vi "Phasor Explorer SEPL Plot Name.vi"(8 "Error In":errorcluster, 11 "Phasor Parameters":T1 {"Detector Parameters"."Frames/Image" min=1; "Detector Parameters"."Multiplicity" min=0; "Detector Parameters"."Bits/Frame" min=1; "Detector Parameters"."Gates/Frame" min=1; "Gate Parameters"."# Steps" min=0.0; "Gate Parameters"."Tolerance" min=0.0; "Gate Parameters"."Top Slope" min=0.0; "Gate Parameters"."Edge Width" min=0.0; "Gate Parameters"."Gate Step" min=0.0; "Gate Parameters"."# Gates" min=0.0 step=1.0; "Gate Parameters"."Gate Width" min=0.0; "Decay & IRF Parameters"."Lifetime" min=0.0; "Decay & IRF Parameters"."IRF Period" min=0.0; "Phasor Parameters"."Square Gate Width" min=0.0; "Phasor Parameters"."# Gates" min=0.0; "Phasor Parameters"."Calibration Lifetime" min=0.0; "Phasor Parameters"."Harmonic Frequency" min=0.0; "Display Parameters"."Min tau" min=0.0; "Display Parameters"."Max tau" min=0.0; "Display Parameters"."# Points" min=1 step=1}) -> (0 "Error Out":errorcluster, 3 "SEPL Plot Name":string)   [LabVIEW 2021, in "Phasor Explorer.lvlib"]
uses:
  Phasor Explorer.lvlib
  Phasor SEPL Parameters.ctl
  Phasor Explorer Display Parameters.ctl
  Phasor Type of Series.ctl
  Phasor Explorer Phasor Parameters.ctl
  Phasor Calculation Type.ctl
  Phasor SEPL Type.ctl
  Phasor Explorer Decay Parameters.ctl
  Phasor IRF Model.ctl
  Phasor Explorer Gate Parameters.ctl
  Phasor Gate Type.ctl
  Phasor Type of User-defined Function.ctl
  Phasor Explorer Detector Parameters.ctl
  Phasor.lvlib
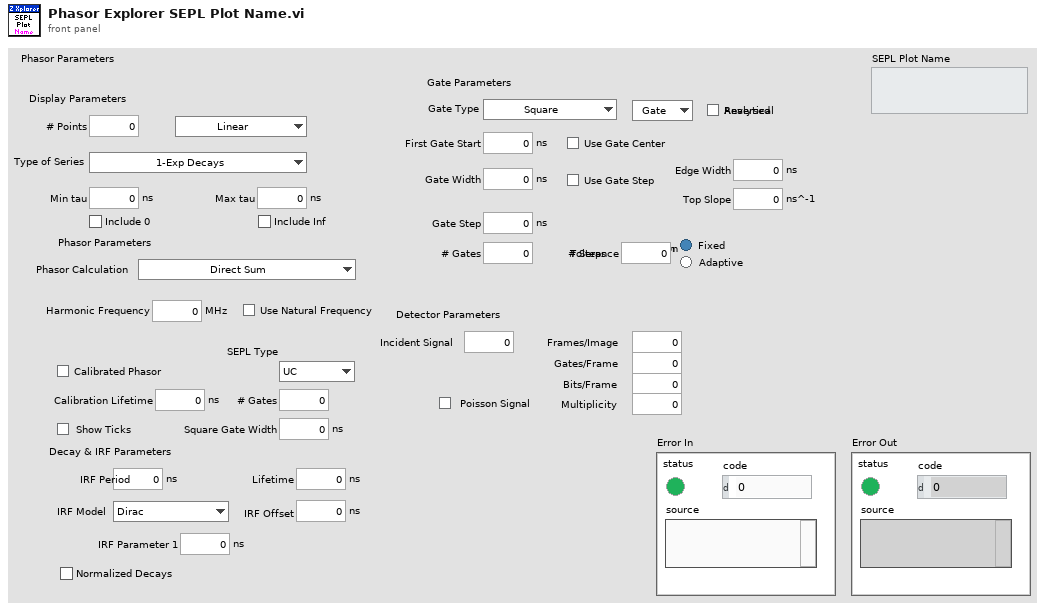
[diagram p1: front panel]
types:
  T1 = typedef "Phasor.lvlib/Phasor SEPL Parameters.ctl" = cluster{"Display Parameters":T2, "Phasor Parameters":T4, "Decay & IRF Parameters":T7, "Gate Parameters":T9, "Detector Parameters":T12}
  T2 = typedef "Phasor Explorer.lvlib/Phasor Explorer Display Parameters.ctl" = cluster{"# Points":i32, "Ramp Type":enum16{"Linear", "Logarithmic"}, "Type of Series":T3, "Min tau":dbl[unit], "Max tau":dbl[unit], "Include 0":bool, "Include Infinity":bool}
  T3 = typedef "Phasor.lvlib/Phasor Type of Series.ctl" = enum16{"1-Exp Decays", "Linear Combination of 1-Exp"}
  T4 = typedef "Phasor Explorer.lvlib/Phasor Explorer Phasor Parameters.ctl" = cluster{"Harmonic Frequency":dbl[unit], "Use f* = 1/D Frequency":bool, "Calibrated Phasor":bool, "Calibration Lifetime":dbl[unit], "Phasor Calculation":T5, "SEPL Type":T6, "# Gates":dbl, "Square Gate Width":dbl[unit], "Show Ticks":bool}
  T5 = typedef "Phasor.lvlib/Phasor Calculation Type.ctl" = enum16{"Direct Sum", "Analytical Formula"}
  T6 = typedef "Phasor.lvlib/Phasor SEPL Type.ctl" = enum16{"UC", "L_N", "L_N[W]", "L_X"}
  T7 = typedef "Phasor Explorer.lvlib/Phasor Explorer Decay Parameters.ctl" = cluster{"Lifetime":dbl[unit], "IRF Offset":dbl[unit], "IRF Period":dbl[unit], "Normalized Decays":bool, "IRF Model":T8, "IRF Parameter 1":dbl[unit]}
  T8 = typedef "Phasor.lvlib/Phasor IRF Model.ctl" = enum16{"Dirac", "Exponential"}
  T9 = typedef "Phasor Explorer.lvlib/Phasor Explorer Gate Parameters.ctl" = cluster{"First Gate Start":dbl[unit], "Use Gate Center":bool, "Gate Width":dbl[unit], "Gate Step":dbl[unit], "# Gates":dbl, "Gate Type":T10, "Edge Width":dbl[unit], "Top Slope":dbl[unit], "Reversed Sawtooth?":bool, "Analytical Computation":bool, "Integration":enum32{"Item 0", "Item 1"}, "Tolerance":dbl, "# Steps":dbl, "Type of User-defined Function":T11, "Use Gate Step":bool}
  T10 = typedef "Phasor.lvlib/Phasor Gate Type.ctl" = enum16{"Square", "Finite Edge Square", "Finite Edge, Tilted Top Square", "Triangle", "Sawtooth", "User-defined"}
  T11 = typedef "Phasor.lvlib/Phasor Type of User-defined Function.ctl" = enum16{"Gate", "IRF"}
  T12 = typedef "Phasor Explorer.lvlib/Phasor Explorer Detector Parameters.ctl" = cluster{"Frames/Image":i32, "Gates/Frame":i32, "Bits/Frame":i32, "Multiplicity":i32, "Incident Signal":dbl, "Poisson Signal":bool}
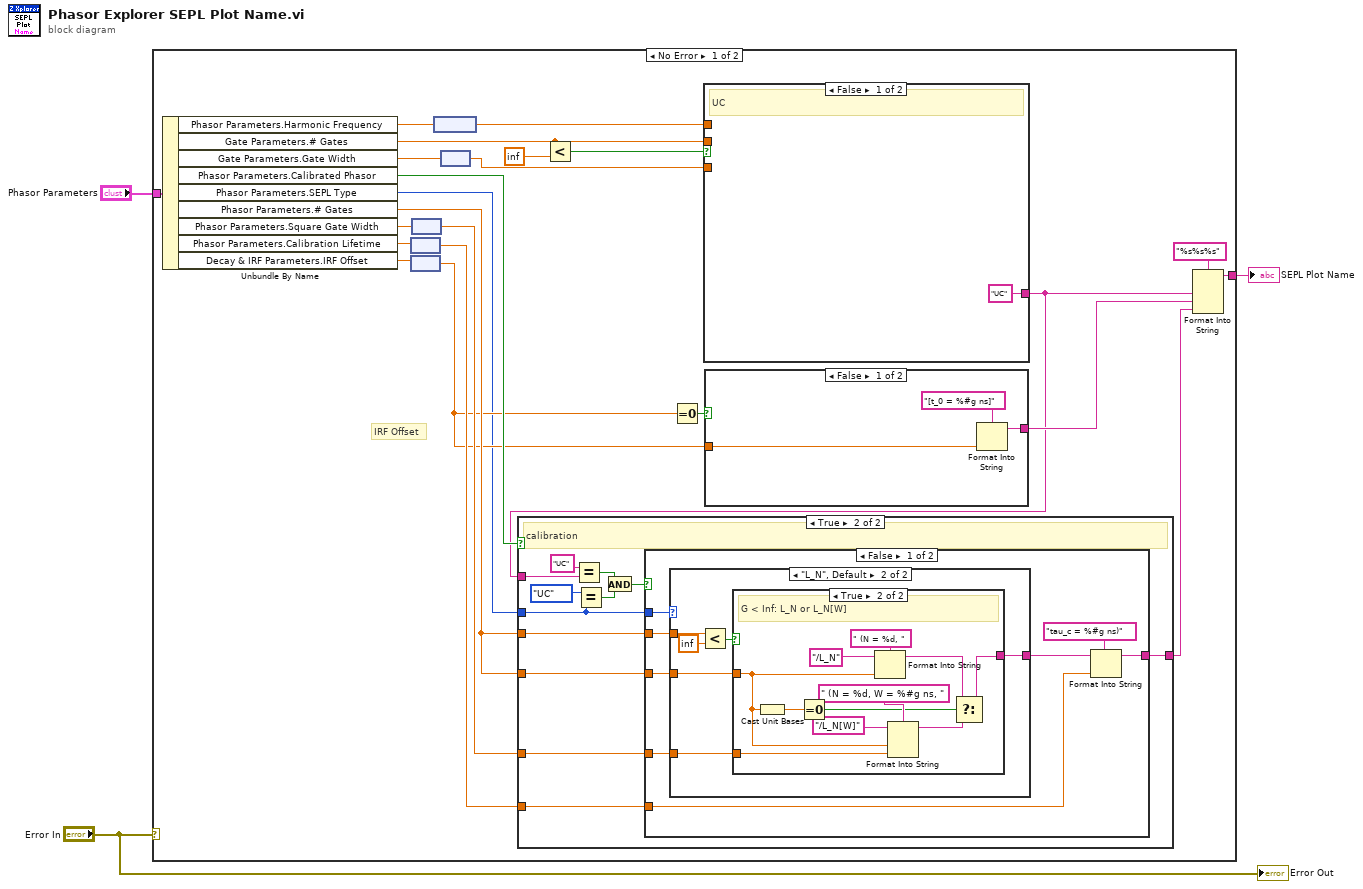
[diagram p0: block diagram]
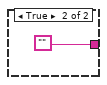
[diagram p2: hidden frame]
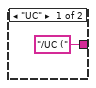
[diagram p4: hidden frame]
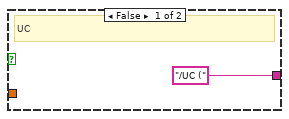
[diagram p5: hidden frame]
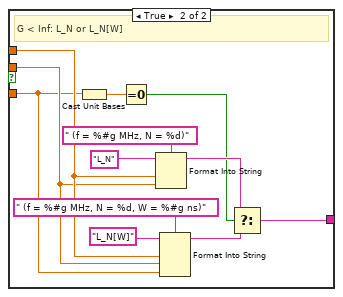
[diagram p7: hidden frame]
diagram:
  n1 = case shown="No Error" "Error In" {
    tunnel: "Phasor Parameters" -> [w25 _]
    tunnel: [w21 _] -> w2
    frame No Error {
      # "IRF Offset"
      n2 = Unbundle By Name(w25) -> ("Phasor Parameters.Harmonic Frequency"=w20:dbl[unit], "Gate Parameters.# Gates"=w19:dbl, "Gate Parameters.Gate Width"=w18:dbl[unit], "Phasor Parameters.Calibrated Phasor"=w17:bool, "Phasor Parameters.SEPL Type"=w5:T6, "Phasor Parameters.# Gates"=w14:dbl, "Phasor Parameters.Square Gate Width"=w16:dbl[unit], "Phasor Parameters.Calibration Lifetime"=w11:dbl[unit], "Decay & IRF Parameters.IRF Offset"=w9:dbl[unit])
      n3 = node(w11) -> (w22:dbl)
      n4 = node(w9) -> (w6:dbl)
      n5 = node(w16) -> (w12:dbl)
      n6 = node(w20) -> (w15:dbl)
      n7 = node(w18) -> (w10:dbl)
      n8 = Less?(x=w19, y=inf) -> (x < y?=w24:bool)
      n9 = Equal To 0?(x=w6) -> (x = 0?=w8:bool)
      n10 = case shown="False" w24 {
        tunnel: ["UC" w82] -> w4
        tunnel: w19 -> [_ w74]
        tunnel: w10 -> [_ w72]
        tunnel: w15 -> [_ w75]
        frame False {
          # "UC"
        }
        frame True {
          # "G < Inf: L_N or L_N[W]"
          n11 = Cast Unit Bases(0:w72) -> (2:w73:dbl)  [unwired: 1 in]
          n12 = Equal To 0?(x=w73) -> (x = 0?=w71:bool)
          n13 = Format Into String(format string=" (f = %#g MHz, N = %d)", initial string="L_N" ("t"), w75, w74) -> (resulting string=w79:string)  [unwired: 1 in, 1 out]
          n14 = Format Into String(format string=" (f = %#g MHz, N = %d, W = %#g ns)", initial string="L_N[W]" ("f"), w75, w74, w72) -> (resulting string=w76:string)  [unwired: 1 in, 1 out]
          n15 = Select(t=w79, s=w71, f=w76) -> (s? t:f=w82:string)
        }
      }
      n16 = case shown="True" w17 {
        tunnel: w22 -> [_ w40]
        tunnel: w14 -> [_ w42]
        tunnel: w14 -> [_ w41]
        tunnel: [_ w39] -> w13
        tunnel: w12 -> [_ w38]
        tunnel: w5 -> [_ w35]
        tunnel: w4 -> [_ w37]
        frame False {
          # "no calibration"
        }
        frame True {
          # "calibration"
          n17 = Equal?(x="UC", y=w37) -> (x = y?=w33:bool)
          n18 = Equal?(x=Phasor_SEPL_Type."UC" ("SEPL Type"), y=w35) -> (x = y?=w32:bool)
          n19 = And(x=w33, y=w32) -> (x .and. y?=w31:bool)
          n20 = case shown="False" w31 {
            tunnel: w42 -> [w50 _]
            tunnel: w41 -> [w49 _]
            tunnel: w40 -> [w47 _]
            tunnel: [w46 _] -> w39
            tunnel: w38 -> [w44 _]
            tunnel: w35 -> [w43 _]
            frame False {
              n21 = case shown="\"L_N\", Default" w43 {
                tunnel: w50 -> [_ w57]
                tunnel: w49 -> [_ w55]
                tunnel: ["/UC (" ("initial string") w53] -> w45
                tunnel: w44 -> [_ w52]
                frame "UC" {
                }
                frame "L_N", Default {
                  n22 = Less?(x=w55, y=inf) -> (x < y?=w54:bool)
                  n23 = case shown="True" w54 {
                    tunnel: w57 -> [_ w61]
                    tunnel: ["/UC (" ("initial string") w59] -> w53
                    tunnel: w52 -> [_ w60]
                    frame False {
                      # "UC"
                    }
                    frame True {
                      # "G < Inf: L_N or L_N[W]"
                      n24 = Cast Unit Bases(0:w61) -> (2:w63:dbl)  [unwired: 1 in]
                      n25 = Equal To 0?(x=w63) -> (x = 0?=w62:bool)
                      n26 = Format Into String(format string=" (N = %d, ", initial string="/L_N" ("t"), w61) -> (resulting string=w67:string)  [unwired: 1 in, 1 out]
                      n27 = Format Into String(format string=" (N = %d, W = %#g ns, ", initial string="/L_N[W]" ("f"), w61, w60) -> (resulting string=w64:string)  [unwired: 1 in, 1 out]
                      n28 = Select(t=w67, s=w62, f=w64) -> (s? t:f=w59:string)
                    }
                  }
                }
              }
              n29 = Format Into String(format string="tau_c = %#g ns)", initial string=w45, w47) -> (resulting string=w46:string)  [unwired: 1 in, 1 out]
            }
            frame True {
            }
          }
        }
      }
      n30 = case shown="False" w8 {
        tunnel: [w29 ""] -> w7
        tunnel: w6 -> [w27 _]
        frame False {
          n31 = Format Into String(format string="[t_0 = %#g ns]", w27) -> (resulting string=w29:string)  [unwired: 2 in, 1 out]
        }
        frame True {
        }
      }
      n32 = Format Into String(format string="%s%s%s", w4, w7, w13) -> (resulting string=w21:string)  [unwired: 2 in, 1 out]
    }
    frame Error {
    }
  }
  "SEPL Plot Name" <- w2
  "Error Out" <- "Error In"
